vi "End.vi"(8 "error in (no error)":errorcluster, 11 "Stream in":refnum<class "Stream.lvclass">) -> (0 "error out":errorcluster, 3 "Stream out":refnum<class "Stream.lvclass">)   [LabVIEW 2018, in "Stream.lvclass"]
uses:
  Stream.lvclass
  Stream.lvclass/Stream.ctl
panel:
  out "error out 3":errorcluster
  out "error out 2":errorcluster
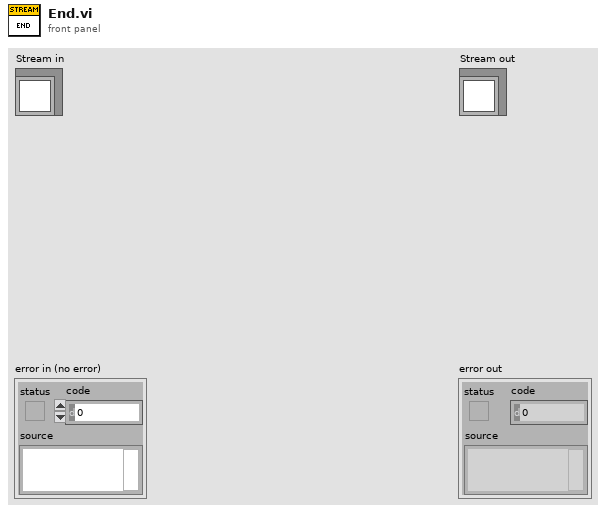
[diagram p1: front panel]
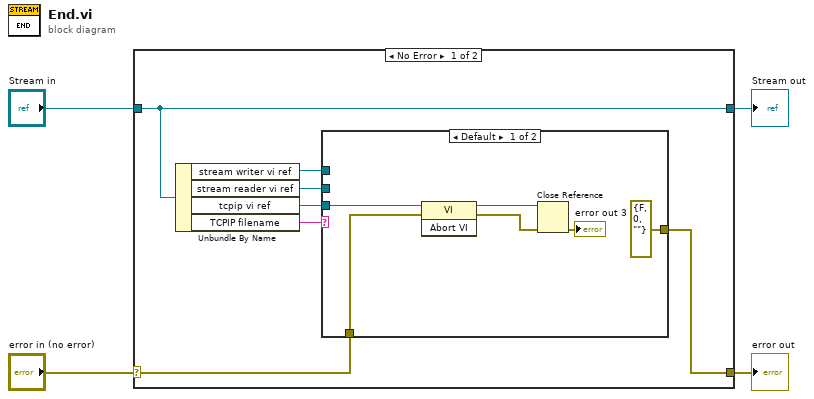
[diagram p0: block diagram]
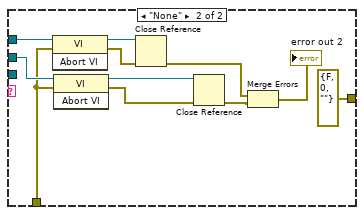
[diagram p2: hidden frame]
diagram:
  n1 = case shown="No Error" "error in (no error)" {
    selector: "error in (no error)" -> [w6 w30]
    tunnel: [w10 w30] -> w3
    tunnel: [w11 w29] -> w1
    tunnel: "Stream in" -> [w11 w29]
    frame No Error {
      n2 = Unbundle By Name(w11) -> ("stream writer vi ref"=w9:refnum<vi>, "stream reader vi ref"=w8:refnum<vi>, "tcpip vi ref"=w7:refnum<vi>, "TCPIP filename"=w5:string)
      n3 = case shown="Default" w5 {
        tunnel: [errorcluster {"status"=FALSE, "code"=0, "source"=""} ("error out") errorcluster {"status"=FALSE, "code"=0, "source"=""} ("error out")] -> w10
        tunnel: w9 -> [_ w28]
        tunnel: w8 -> [_ w26]
        tunnel: w7 -> [w16 _]
        tunnel: w6 -> [w15 w22]
        frame Default {
          n4 = invoke class="VI" method="Abort VI"(reference=w16, error in=w15) -> (reference out=w17:refnum<vi>, error out=w14:errorcluster)  [unwired: 1 in, 1 out]
          n5 = Close Reference(reference=w17, error in (no error)=w14) -> (error out=→"error out 3":errorcluster)
        }
        frame "None" {
          n6 = invoke class="VI" method="Abort VI"(reference=w28, error in=w22) -> (reference out=w27:refnum<vi>, error out=w24:errorcluster)  [unwired: 1 in, 1 out]
          n7 = invoke class="VI" method="Abort VI"(reference=w26, error in=w22) -> (reference out=w25:refnum<vi>, error out=w23:errorcluster)  [unwired: 1 in, 1 out]
          n8 = Close Reference(reference=w27, error in (no error)=w24) -> (error out=w20:errorcluster)
          n9 = Close Reference(reference=w25, error in (no error)=w23) -> (error out=w19:errorcluster)
          n10 = Merge Errors(w20, w19) -> (→"error out 2":errorcluster)
        }
      }
    }
    frame Error {
    }
  }
  "error out" <- w3
  "Stream out" <- w1
